vi "LINX_PC.vi"() -> ()   [LabVIEW 2014]
uses:
  <vilib>/MakerHub/LINX/Private/Device/Type Defs/TCP Config.ctl
  <vilib>/MakerHub/LINX/Public/Utilities/Open TCP.vi
  <vilib>/MakerHub/LINX/LMH-LINX.lvlib
  <vilib>/MakerHub/LINX/Private/Device/Device.lvlib
panel:
  in  "stop":bool
  out "Waveform Chart":dbl[](graph)
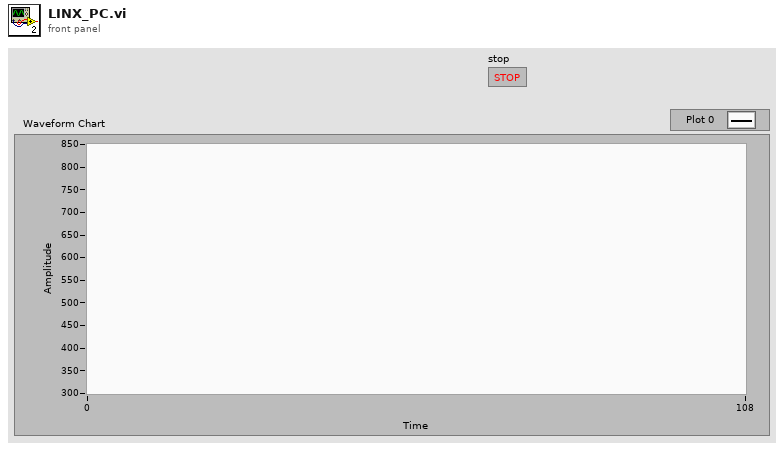
[diagram p1: front panel]
types:
  T1 = typedef "LMH-LINX.lvlib/Device.lvlib/TCP Config.ctl" = cluster{"IP Address":string, "Port":u16}
  T2 = cluster{"ADS1015-Channel Selector":enum8{"DIFF-AI0-AI1", "DIFF-AI0-AI3", "DIFF-AI1-AI3", "DIFF-AI2-AI3", "Single Ended - AI0", "Single Ended - AI1", "Single Ended - AI2", "Single Ended - AI3"}, "ADS1015 -Gain & Scale":enum8{"FS=+/-6.144 V", "FS=+/-4.096 V", "FS=+/-2.048 V", "FS=+/-1.024 V", "FS=+/-0.512 V", "FS=+/-0.256-A V", "FS=+/-0.256-B V", "FS=+/-0.256-C V"}, "ADS1015- Acquire Mode":enum16{"Continuous Conversion Mode", "Single Shot Mode"}, "ADS1015 Sample Rate":enum8{"128 SPS", "250 SPS", "490 SPS", "920 SPS", "1600 SPS", "2400 SPS", "3300 SPS", "3300 SPS A"}}
  T3 = typedef "LMH-LINX.lvlib/LINX Ref.ctl" = cluster{"IO":T4, "Interface":T5, "LINX Device Config":T6}
  T4 = typedef "LMH-LINX.lvlib/Platform.ctl" = enum16{"Remote", "Local"}
  T5 = typedef "LMH-LINX.lvlib/Interface.ctl" = enum16{"Serial", "TCP"}
  T6 = typedef "LMH-LINX.lvlib/Device.lvlib/LINX Device Config.ctl" = cluster{"Interface":T5, "COM Port":refnum<visa-resource-name>, "TCP Configuration":T1, "Device Family":u8, "Device ID":u8, "Device Name":string, "TCP Ref":refnum<k5>, "Channels":T7}
  T7 = typedef "LMH-LINX.lvlib/Channels.ctl" = cluster{"DI":u8[], "DO":u8[], "AI":u8[], "AO":u8[], "PWM":u8[], "QE":u8[], "UART":u8[], "I2C 2":u8[], "SPI":u8[], "CAN":u8[], "Servo":u8[], "AI Ref (V)":dbl, "AI Resolution (Bits)":u8, "AO Ref (V)":dbl, "AO Resolution (Bits)":u8}
  T8 = enum8{"FS=+/-6.144 V", "FS=+/-4.096 V", "FS=+/-2.048 V", "FS=+/-1.024 V", "FS=+/-0.512 V", "FS=+/-0.256-A V", "FS=+/-0.256-B V", "FS=+/-0.256-C V"}
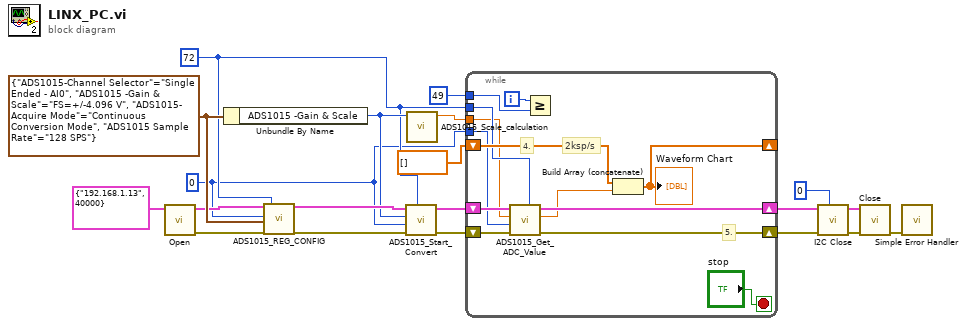
[diagram p0: block diagram]
diagram:
  w1 = u8 0 ("I2C Channel (RPI)")
  w3 = u8 72 ("I2C Slave Address (0)")
  w13 = T2 {"ADS1015-Channel Selector"=enum."Single Ended - AI0", "ADS1015 -Gain & Scale"=enum."FS=+/-4.096 V", "ADS1015- Acquire Mode"=enum."Continuous Conversion Mode", "ADS1015 Sample Rate"=enum."128 SPS"} ("ADS1015 Reg Config")
  n1 = call-poly <vilib>:"Open.vi"("TCP Configuration"=T1 {"IP Address"="192.168.1.13", "Port"=40000}) -> ("Error Out"=w4:errorcluster, "LINX Resource"=w5:T3)  [unwired: 8 in, 1 out]
  n2 = Unbundle By Name(w13) -> ("ADS1015 -Gain & Scale"=w12:T8)
  n3 = call "ADS1015_REG_CONFIG.vi"("LINX Resource in"=w5, "I2C Channel (RPI)"=w1, "ADS1015 Reg Config"=w13, "Error In"=w4, "I2C Slave Address (0)"=w3) -> ("LINX Resource out"=w16:T3, "Error Out"=w19:errorcluster)  [unwired: 13 in]
  n4 = call "ADS1015_Start_Convert.vi"("I2C Slave Address (0)"=w3, "error in (no error)"=w19, "I2C Channel (RPI)"=w1, "Scale mV"=w12, "LINX Resource in"=w16) -> ("error out"=w18:errorcluster, "LINX Resource out"=w15:T3)  [unwired: 4 in, 1 out]
  n5 = call "ADS1015_Scale_calculation.vi"("ADS1015 -Gain & Scale"=w12) -> ("Scale Value (mV)"=w14:dbl)  [unwired: 10 in]
  n6 = while {
    shift-right: [w28] -> w10
    shift-left: w15 -> [w29]
    shift-right: [w33] -> w8
    shift-left: w18 -> [w32]
    shift-right: [w23] -> _
    shift-left: dbl[] [] -> [w31]
    tunnel: w3 -> [w27]
    tunnel: w14 -> [w25]
    tunnel: 49 ("y") -> [w24]
    tunnel: w1 -> [w21]
    i -> [w30]
    stop <- "stop" stop-if-true
    # "2ksp/s"
    # "5."
    # "4."
    n7 = call "ADS1015_Get_ADC_Value.vi"("I2C Slave Address (0)"=w27, "error in (no error)"=w32, "I2C Channel (RPI)"=w21, "Scale Value (mV)"=w25, "LINX Resource in"=w29) -> ("error out"=w33:errorcluster, "mV out"=w26:dbl, "LINX Resource"=w28:T3)  [unwired: 4 in]
    n8 = Greater Or Equal?(x=w30, y=w24) -> ()  [unwired: 1 out]
    n9 = Build Array (concatenate)(w31, w26) -> (w23:dbl[])
    "Waveform Chart" <- w23
  }
  n10 = call <vilib>:"I2C Close.vi"("I2C Channel (0)"=u8 0, "Error In"=w8, "LINX Resource"=w10) -> ("Error Out"=w7:errorcluster, "LINX Resource"=w9:T3)  [unwired: 7 in]
  n11 = call <vilib>:"Close.vi"("Error In"=w7, "LINX Resource"=w9) -> ("Error Out"=w20:errorcluster)  [unwired: 9 in]
  n12 = call <vilib>:"Simple Error Handler.vi"("error in (no error)"=w20) -> ()  [unwired: 4 in, 5 out]
